vi "SMO.UI.Splash.TestLauncher.vi"() -> ()   [LabVIEW 2013, in "SMO.UI.Splash.lvclass"]
doc: "JKI State Machine Objects (SMO) 1.0.0.5\nJKI - JKI\nCopyright (c) 2016, JKI"
uses:
  SMO.UI.Splash.lvclass
  <vilib>/JKI/JKI SMO/SMO/SMO.lvclass
  <vilib>/JKI/JKI SMO/SMO.UI/SMO.UI.lvclass
panel:
  out "error out":errorcluster
  in  "Stop":bool
  # "SMO Splash Test Launcher"
  # "For instructions on how to use the JKI State Machine Objects, examples and video tutorials, visit:\nhttp://jki.net/state-machine-objects/\n\nJKI State Machine Objects™\nhttp://jki.net/state-machine-objects/\nCopyright (C) 2005-2015, JKI <info@jki.net>\nALL RIGHTS RESERVED"
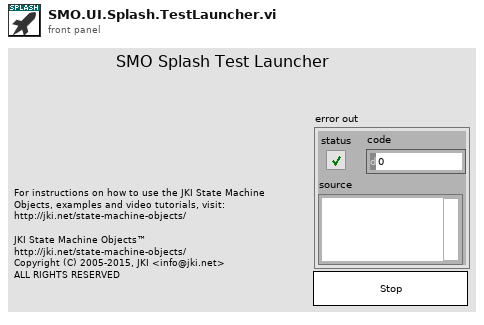
[diagram p1: front panel]
types:
  T1 = typedef "SMO.UI.lvclass/PublicEvents--Cluster.ctl" = cluster{"UI Hidden":refnum<user-event>, "UI State":refnum<user-event>}
  T2 = cluster{"Event Registration Refnum":refnum<event-registration>}
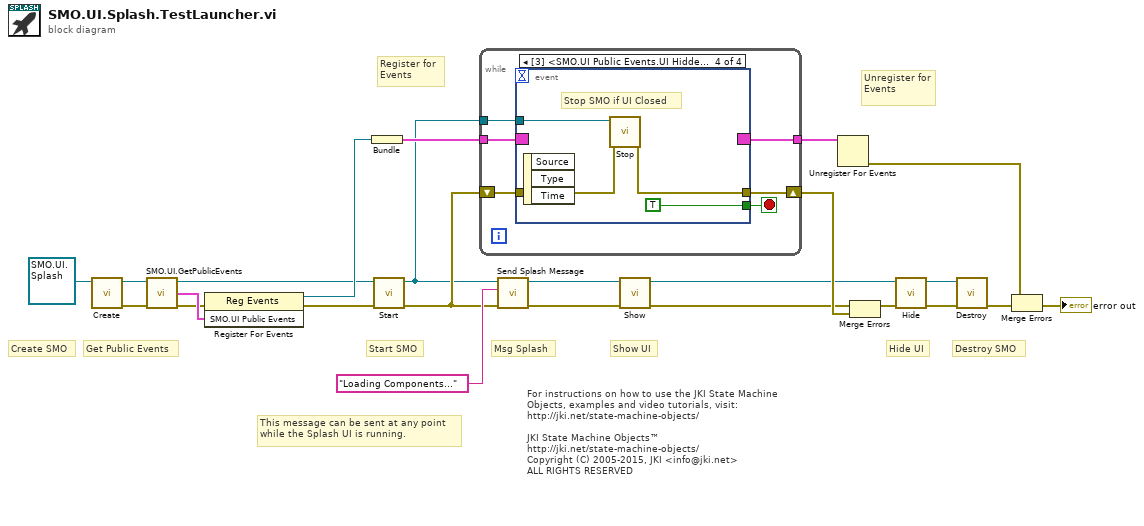
[diagram p0: block diagram]
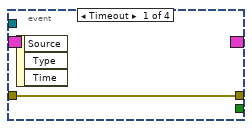
[diagram p2: hidden frame]
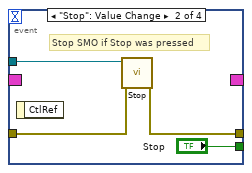
[diagram p3: hidden frame]
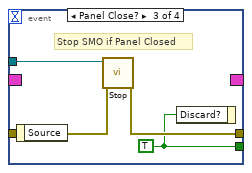
[diagram p4: hidden frame]
diagram:
  # "Msg Splash"
  # "This message can be sent at any point\nwhile the Splash UI is running."
  # "Hide UI"
  # "Show UI"
  # "For instructions on how to use the JKI State Machine Objects, examples and video tutorials, visit:\nhttp://jki.net/state-machine-objects/\n\nJKI State Machine Objects™\nhttp://jki.net/state-machine-objects/\nCopyright (C) 2005-2015, JKI <info@jki.net>\nALL RIGHTS RESERVED"
  # "Get Public Events"
  # "Start SMO"
  # "Destroy SMO"
  # "Create SMO"
  # "Unregister for Events"
  # "Register for Events"
  n1 = call <vilib>:"Create.vi"("SMO"=refnum<class "SMO.UI.Splash.lvclass"> refnum ("SMO.Template.lvclass")) -> ("error out"=w3:errorcluster, "SMO out"=w5:refnum<class "SMO.UI.Splash.lvclass">)  [unwired: 8 in, 1 out]
  n2 = call <vilib>:"SMO.UI.GetPublicEvents.vi"("error in (no error)"=w3, "SMO.UI"=w5) -> ("error out"=w6:errorcluster, "SMO.UI Public Events"=w7:T1, "SMO.UI out"=w1:refnum<class "SMO.UI.Splash.lvclass">)  [unwired: 7 in]
  n3 = register-events(error in=w6, w7) -> (reference out=w4:refnum<event-registration>, error out=w2:errorcluster)  [unwired: 1 in]
  n4 = Bundle("Event Registration Refnum"=w4) -> (w23:T2)  [unwired: 1 in]
  n5 = call <vilib>:"Start.vi"("error in (no error)"=w2, "SMO"=w1) -> ("error out"=w11:errorcluster, "SMO out"=w8:refnum<class "SMO.UI.Splash.lvclass">)  [unwired: 8 in]
  n6 = while {
    shift-right: [w29] -> w22
    shift-left: w11 -> [w28]
    tunnel: w23 -> [w27]
    tunnel: [w26] -> w24
    tunnel: w8 -> [w25]
    stop <- w30 stop-if-true
    n7 = event shown="[3] <SMO.UI Public Events.UI Hidden>: User Event" {
      selector: w27 -> [_ _ _ _]
      dyn-events: [_ _ _ _] -> w26
      timeout: _ -> [_ _ _ _]
      tunnel: [_ "Stop" w36 TRUE ("OK")] -> w30
      tunnel: w25 -> [_ w33 w39 w43]
      tunnel: [w31 w34 w38 w42] -> w29
      tunnel: w28 -> [w31 w32 w37 w41]
      event Timeout {
        n8 = event-data() -> ()  [unwired: 1 in, 3 out]
      }
      event "Stop": Value Change {
        # "Stop SMO if Stop was pressed"
        n9 = event-data() -> ()  [unwired: 1 in, 1 out]
        n10 = call <vilib>:"Stop.vi"("error in (no error)"=w32, "SMO"=w33) -> ("error out"=w34:errorcluster)  [unwired: 8 in, 1 out]
      }
      event Panel Close? {
        w36 = TRUE ("OK")
        # "Stop SMO if Panel Closed"
        n11 = event-data() -> ()  [unwired: 1 in, 1 out]
        n12 = call <vilib>:"Stop.vi"("error in (no error)"=w37, "SMO"=w39) -> ("error out"=w38:errorcluster)  [unwired: 8 in, 1 out]
        n13 = event-data("Discard?"=w36) -> ()  [unwired: 1 in, 1 out]
      }
      event User Event {
        # "Stop SMO if UI Closed"
        n14 = event-data() -> ()  [unwired: 1 in, 3 out]
        n15 = call <vilib>:"Stop.vi"("error in (no error)"=w41, "SMO"=w43) -> ("error out"=w42:errorcluster)  [unwired: 8 in, 1 out]
      }
    }
  }
  n16 = call-dynamic "Send Splash Message.vi"("error in (no error)"=w11, "Message"="Loading Components...", "SMO.UI.Splash in"=w8) -> ("error out"=w10:errorcluster, "SMO.UI.Splash out"=w9:refnum<class "SMO.UI.Splash.lvclass">)  [unwired: 7 in]
  n17 = call <vilib>:"Show.vi"("error in (no error)"=w10, "SMO.UI"=w9) -> ("error out"=w17:errorcluster, "SMO.UI out"=w16:refnum<class "SMO.UI.Splash.lvclass">)  [unwired: 8 in]
  n18 = Unregister For Events(event registration refnum=w24) -> (error out=w21:errorcluster)  [unwired: 1 in]
  n19 = Merge Errors(w17, w22) -> (w14:errorcluster)
  n20 = call <vilib>:"Hide.vi"("error in (no error)"=w14, "SMO.UI"=w16) -> ("error out"=w13:errorcluster, "SMO.UI out"=w15:refnum<class "SMO.UI.Splash.lvclass">)  [unwired: 8 in]
  n21 = call <vilib>:"Destroy.vi"("error in (no error)"=w13, "SMO"=w15) -> ("error out"=w19:errorcluster)  [unwired: 9 in]
  n22 = Merge Errors(w21, w19) -> (→"error out":errorcluster)
